vi "LogWrite.vi"   [LabVIEW 2019]
uses:
  <vilib>/Utility/file.llb/Write Delimited Spreadsheet (string).vi
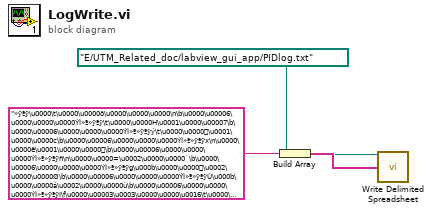
[diagram p0: block diagram]
diagram:
  n1 = Build Array("»ÿªÿ\u0000\t\u0000\u0000ö\u0000\u0000\u0000\n\b\u0000\u00006\u0000\u0000\u0000ÝÌ»ª»ÿªÿ\t\u0000\u0000H\u0001\u0000\u00007\b\u0000\u00006\u0000\u0000\u0000ÝÌ»ª»ÿªÿý\t\u0000\u0000\u0001\u0000\u0000c\b\u0000\u00006\u0000\u0000\u0000ÝÌ»ª»ÿªÿx\n\u0000\u0000ë\u0001\u0000\u0000\b\u0000\u00006\u0000\u0000\u0000ÝÌ»ª»ÿªÿñ\n\u0000\u0000=\u0002\u0000\u0000´\b\u0000\u00006\u0000\u0000\u0000ÝÌ»ª»ÿªÿg\u000b\u0000\u0000\u0002\u0000\u0000Ø\b\u0000\u00006\u0000\u0000\u0000ÝÌ»ª»ÿªÿÚ\u000b\u0000\u0000á\u0002\u0000\u0000ù\b\u0000\u00006\u0000\u0000\u0000ÝÌ»ª»ÿªÿI\f\u0000\u00003\u0003\u0000\u0000\u0016\t\u0000\u00006\u0000\u0000\u0000ÝÌ»ª»ÿªÿ³\f\u0000\u0000\u0003\u0000\u0000.\t\u0000\u00006\u0000\u0000\u0000ÝÌ»ª»ÿªÿ\u0019\r\u0000\u0000×\u0003\u0000\u0000B\t\u0000\u00006\u0000\u0000\u0000ÝÌ»ª»ÿªÿy\r\u0000\u0000)\u0004\u0000\u0000P\t\u0000\u00006\u0000\u0000\u0000ÝÌ»ª»ÿªÿÔ\r\u0000\u0000{\u0004\u0000\u0000Y\t\u0000\u00006\u0000\u0000\u0000ÝÌ»ª»ÿªÿ)\u000e\u0000\u0000Í\u0004\u0000\u0000\\\t\u0000\u00006\u0000\u0000\u0000ÝÌ»ª»ÿªÿx\u000e\u0000\u0000\u001e\u0005\u0000\u0000Z\t\u0000\u00006\u0000\u0000\u0000ÝÌ»ª»ÿªÿÀ\u000e\u0000\u0000p\u0005\u0000\u0000P\t\u0000\u00006\u0000\u0000\u0000ÝÌ»ª»ÿªÿ\u0002\u000f\u0000\u0000Â\u0005\u0000\u0000@\t\u0000\u00006\u0000\u0000\u0000ÝÌ»ª»ÿªÿ<\u000f\u0000\u0000\u0014\u0006\u0000\u0000(\t\u0000\u00006\u0000\u0000\u0000ÝÌ»ª»ÿªÿo\u000f\u0000\u0000f\u0006\u0000\u0000\t\t\u0000\u00006\u0000\u0000\u0000ÝÌ»ª»ÿªÿ\u000f\u0000\u0000¸\u0006\u0000\u0000ã\b\u0000\u00006\u0000\u0000\u0000ÝÌ»ª»ÿªÿ¿\u000f\u0000\u0000\n\u0007\u0000\u0000µ\b\u0000\u00006\u0000\u0000\u0000ÝÌ»ª»ÿªÿÛ\u000f\u0000\u0000\\\u0007\u0000\u0000\b\u0000\u00006\u0000\u0000\u0000ÝÌ»ª»ÿªÿï\u000f\u0000\u0000®\u0007\u0000\u0000A\b\u0000\u00006\u0000\u0000\u0000ÝÌ»ª»ÿªÿû\u000f\u0000\u0000\u0000\b\u0000\u0000û\u0007\u0000\u00006\u0000\u0000\u0000ÝÌ»ª»ÿªÿÿ\u000f\u0000\u0000Q\b\u0000\u0000®\u0007\u0000\u00006\u0000\u0000\u0000ÝÌ»ª»ÿªÿû\u000f\u0000\u0000£\b\u0000\u0000X\u0007\u0000\u00006\u0000\u0000\u0000ÝÌ»ª...") -> (w2:string[])
  n2 = call-poly <vilib>:"Write Delimited Spreadsheet.vi"("file path (dialog if empty)"=path "E:/UTM_Related_doc/labview_gui_app/PIDlog.txt", "1D data"=w2) -> ()  [unwired: 12 in, 2 out]
